vi "create_try.vi"() -> ()   [LabVIEW 2013]
panel:
  out "UID":i32
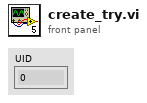
[diagram p1: front panel]
types:
  T1 = enum8{"Probe", "Diagram", "Panel Control", "3D Panel Control", "Dialog Panel Control", "Panel Indicator", "3D Panel Indicator", "Dialog Panel Indicator", "Power PC Control", "Power PC Indicator", "Silver Control", "Silver Indicator"}
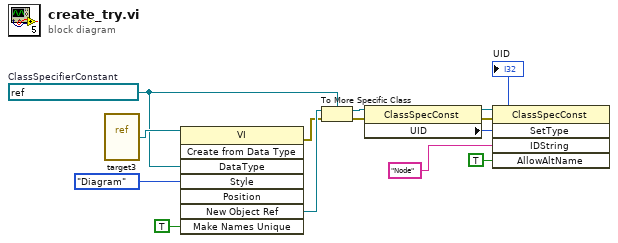
[diagram p0: block diagram]
diagram:
  w7 = refnum<vi> refnum  # ClassSpecifierConstant
  n1 = vi-ref "target3.vi"() -> (w12:refnum<vi>)
  n2 = invoke class="VI" method="Create from Data Type"(reference=w12, "DataType"=w7, "Style"=T1."Diagram", "Make Names Unique"=TRUE ("Make Names Unique (F)")) -> (error out=w6:errorcluster, "New Object Ref"=w8:refnum<vi>)  [unwired: 4 in, 6 out]
  n3 = To More Specific Class(target class=w7, reference=w8, error in=w6) -> (specific class reference=w5:refnum<vi>, error out=w4:errorcluster)
  n4 = property class="ClassSpecConst"(reference=w5, error in=w4) -> (reference out=w10:refnum<vi>, error out=w9:errorcluster, "UID"=→"UID":i32)
  n5 = invoke class="ClassSpecConst" method="SetType"(reference=w10, error in=w9, "IDString"="Node" ("ID String"), "AllowAltName"=TRUE ("Allow Alternate Name? (F)")) -> ()  [unwired: 1 in, 5 out]
